vi "Main.vi"(8 "error in":errorcluster, 11 "TCP Receive in":refnum<class "TCP Receive.lvclass">) -> (0 "error out":errorcluster, 3 "TCP Receive out":refnum<class "TCP Receive.lvclass">)   [LabVIEW 2020, in "TCP Receive.lvclass"]
doc: "The Queued Message Handler of a Worker."
uses:
  TCP Receive.lvclass
  C:/Program Files (x86)/National Instruments/LabVIEW 2020/vi.lib/addons/_Workers/Library/Classes/Worker/Worker.lvclass
  Initialization Data.ctl
  <vilib>/addons/_Workers/Library/Classes/Message Queue/Message Queue.lvclass
  TCP Receive.lvclass/TCP Receive.ctl
  <vilib>/addons/_Workers/Library/Classes/Message/Enqueue Message to Self.vi
  <vilib>/addons/_Workers/Library/Classes/Message/Enqueue Message to Queue.vi
  <vilib>/addons/_Workers/Library/Classes/EHL/EHL.lvclass
  <vilib>/addons/_Workers/Library/Classes/Worker/Worker.lvclass
  <vilib>/addons/_Workers/Library/Classes/Error Handler/Error Handler.lvclass
  C:/Program Files (x86)/National Instruments/LabVIEW 2020/vi.lib/addons/_Workers/Library/Classes/Worker User/Worker User.lvclass
  C:/Program Files (x86)/National Instruments/LabVIEW 2020/vi.lib/addons/_Workers/Library/Classes/Workers Object/Workers Object.lvclass
  C:/Users/TestAdmin/git/TCP-Workers/Workers/TCP Receive/TCP Receive.lvclass
  <vilib>/addons/_Workers/Library/Classes/Message/Message.lvclass
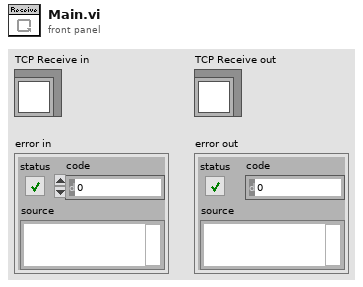
[diagram p1: front panel]
types:
  T1 = typedef "TCP Receive.lvclass/Initialization Data.ctl" = cluster{"String":string, "connection ID":refnum<k5>, "End Point":refnum<class "Message Queue.lvclass">}
  T2 = enum16{"Standard", "Buffered", "CRLF", "Immediate"}
  T3 = typedef "Workers.lvlib/Case Label.ctl" = string
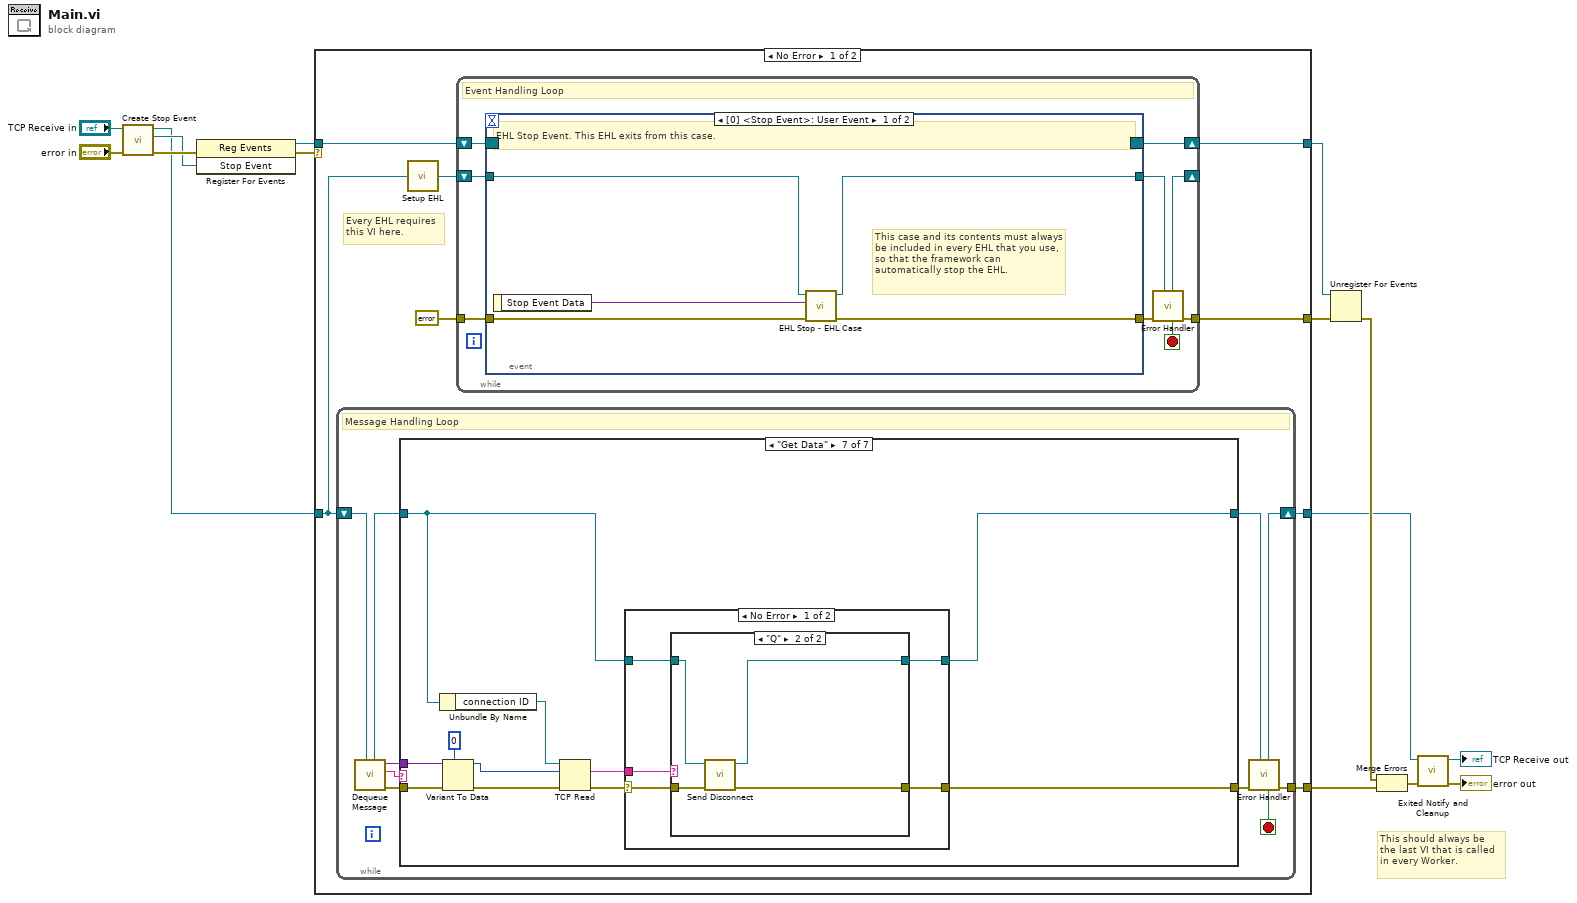
[diagram p0: block diagram]
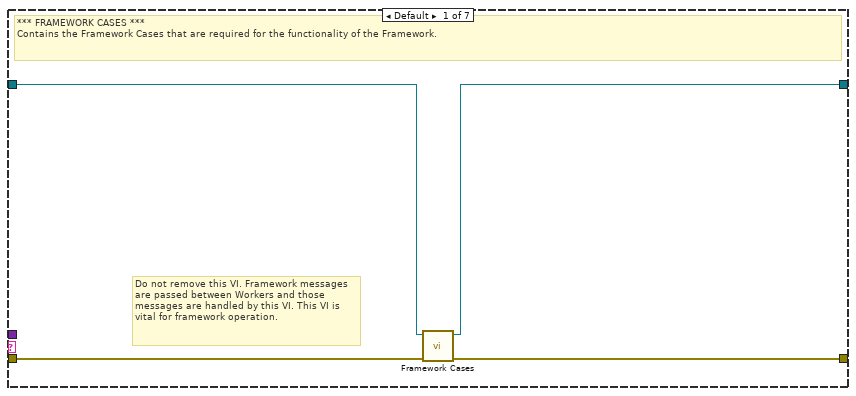
[diagram p2: hidden frame]
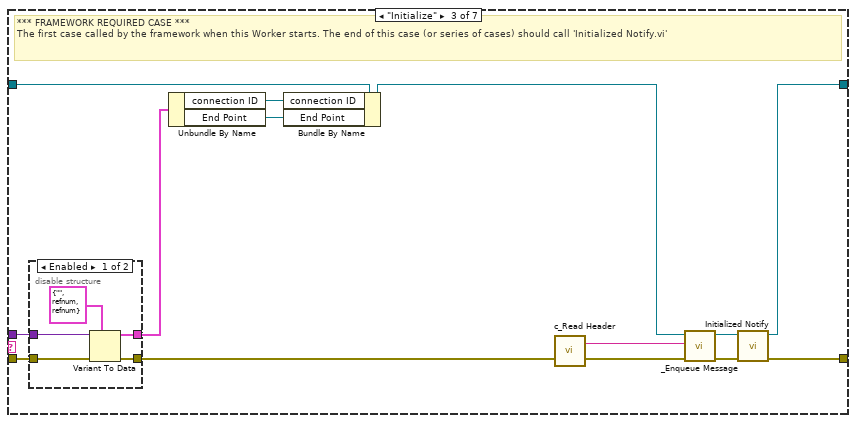
[diagram p4: hidden frame]
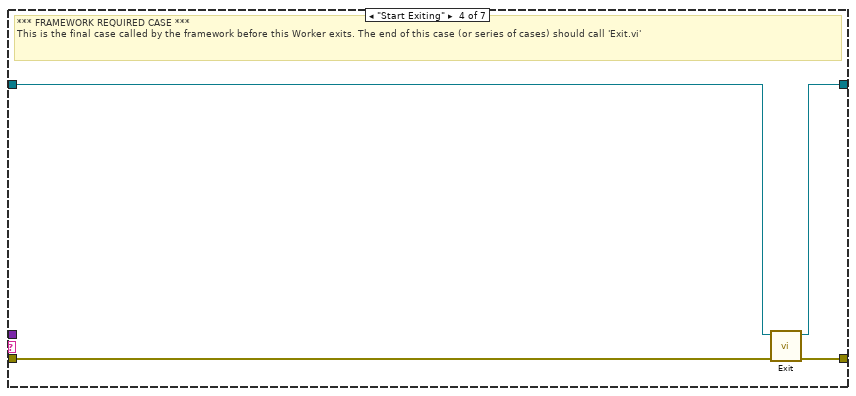
[diagram p6: hidden frame]
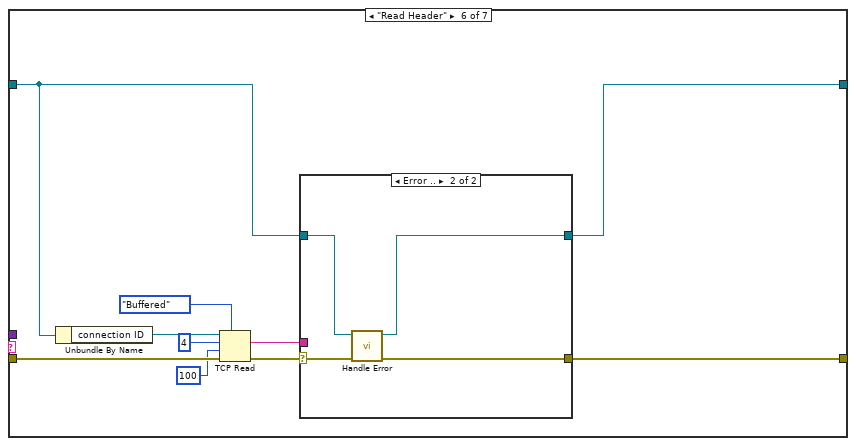
[diagram p8: hidden frame]
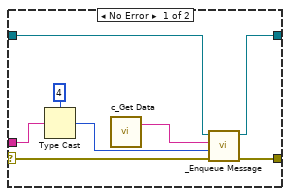
[diagram p9: hidden frame]
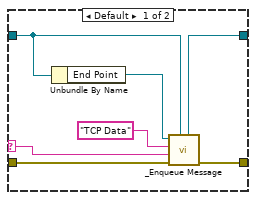
[diagram p10: hidden frame]
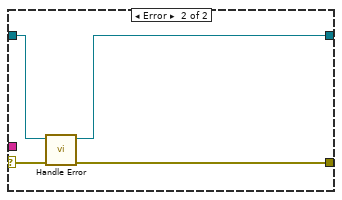
[diagram p11: hidden frame]
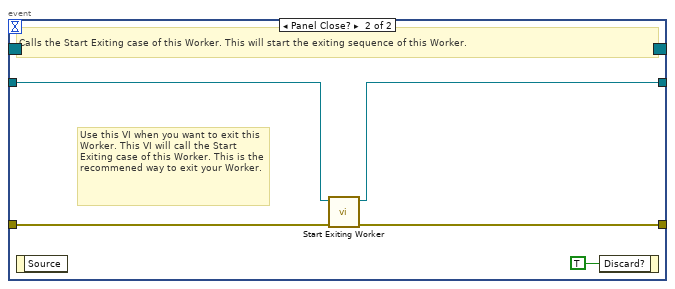
[diagram p12: hidden frame]
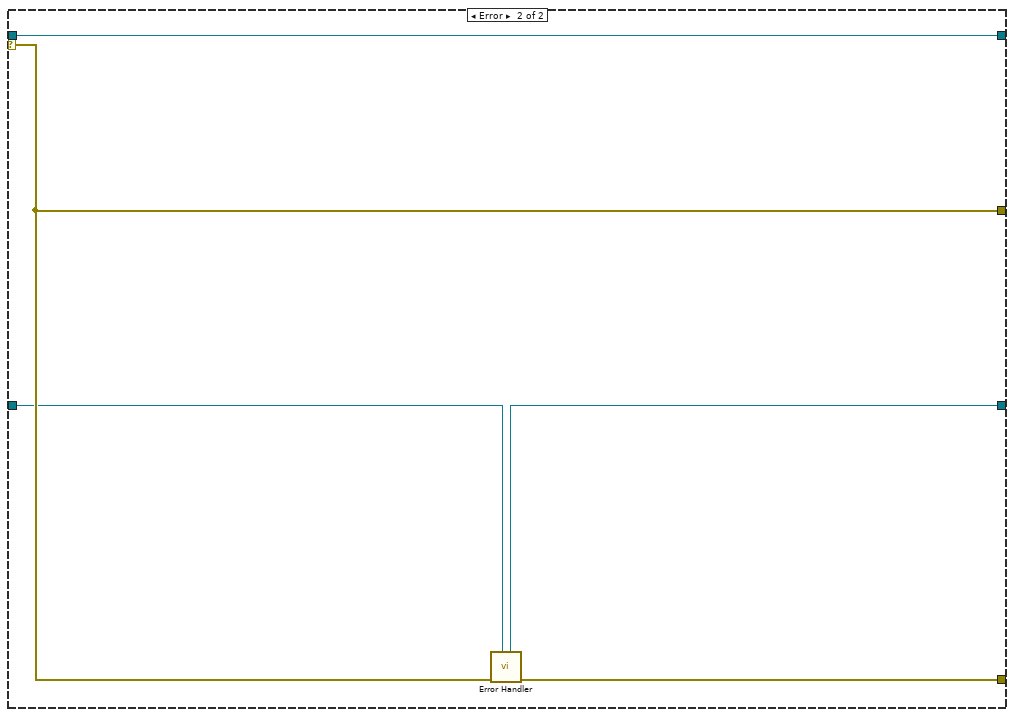
[diagram p13: hidden frame]
diagram:
  # "This should always be the last VI that is called in every Worker."
  n1 = call <vilib>:"Create Stop Event.vi"("error in"="error in", "Worker"="TCP Receive in") -> ("error out"=w10:errorcluster, "Stop Event"=w7:refnum<user-event>, "Worker out"=w4:refnum<class "TCP Receive.lvclass">)  [unwired: 7 in]
  n2 = register-events(error in=w10, w7) -> (reference out=w9:refnum<event-registration>, error out=w1:errorcluster)  [unwired: 1 in]
  n3 = case shown="No Error" w1 {
    tunnel: w4 -> [w18 w138]
    tunnel: [w16 w139] -> w8
    tunnel: w9 -> [w23 w140]
    tunnel: [w20 w141] -> w14
    tunnel: [w22 w140] -> w13
    tunnel: [w17 w137] -> w11
    selector: w1 -> [_ w141]
    frame No Error {
      # "Every EHL requires\nthis VI here."
      n4 = while {
        shift-right: [w31] -> w17
        shift-left: w18 -> [w33]
        tunnel: [w32] -> w16
        stop <- w24 stop-if-true
        # "Message Handling Loop"
        n5 = call <vilib>:"Dequeue Message.vi"("Worker"=w33) -> ("error out"=w30:errorcluster, "Case out"=w25:string, "Data out"=w26:variant, "Worker out"=w28:refnum<class "TCP Receive.lvclass">)  [unwired: 6 in, 1 out]
        n6 = case "WORKERS MHL Case Structure (DO NOT CHANGE LABEL NAME)" shown="\"Get Data\"" w25 {
          tunnel: w30 -> [w37 w38 w50 w59 w63 w74 w97]
          tunnel: [w36 w38 w52 w62 w63 w67 w88] -> w29
          tunnel: w28 -> [w35 w39 w49 w60 w64 w66 w89]
          tunnel: [w34 w39 w51 w61 w64 w65 w87] -> w27
          tunnel: w26 -> [_ _ w47 _ _ _ w95]
          frame Default {
            # "Do not remove this VI. Framework messages are passed between Workers and those messages are handled by this VI. This VI is vital for framework operation."
            # "*** FRAMEWORK CASES ***\nContains the Framework Cases that are required for the functionality of the Framework."
            n7 = call <vilib>:"Framework Cases.vi"("error in"=w37, "Worker"=w35) -> ("error out"=w36:errorcluster, "Worker out"=w34:refnum<class "TCP Receive.lvclass">)  [unwired: 8 in]
          }
          frame "------ FRAMEWORK REQUIRED CASES ------" {
            # "Start of Framework Required Cases"
          }
          frame "Initialize" {
            # "*** FRAMEWORK REQUIRED CASE ***\nThe first case called by the framework when this Worker starts. The end of this case (or series of cases) should call 'Initialized Notify.vi'"
            n8 = disable-structure shown="Enabled" {
              disable-tunnel: w50 -> [w57 w58]
              disable-tunnel: [w56 w58] -> w48
              disable-tunnel: w47 -> [w55 _]
              disable-tunnel: [w53 _] -> w46
              frame Enabled {
                n9 = Variant To Data(error in=w57, type=T1 {"String"="", "connection ID"=refnum, "End Point"=refnum} ("Initialization Data"), Variant=w55) -> (data=w53:T1, error out=w56:errorcluster)
              }
              frame Disabled {
              }
            }
            n10 = Unbundle By Name(w46) -> ("connection ID"=w45:refnum<k5>, "End Point"=w44:refnum<class "Message Queue.lvclass">)
            n11 = Bundle By Name(cluster=w49, "connection ID"=w45, "End Point"=w44) -> (w42:refnum<class "TCP Receive.lvclass">)
            n12 = call "c_Read Header.vi"() -> ("Case Label"=w40:T3)  [unwired: 1 in]
            n13 = call-poly <vilib>:"_Enqueue Message.vi"("error in"=w48, "Case Label"=w40, "Worker"=w42) -> ("error out"=w43:errorcluster, "dup Worker out"=w41:refnum<class "TCP Receive.lvclass">)  [unwired: 7 in]
            n14 = call <vilib>:"Initialized Notify.vi"("error in"=w43, "Worker"=w41) -> ("error out"=w52:errorcluster, "dup Worker out"=w51:refnum<class "TCP Receive.lvclass">)  [unwired: 8 in]
          }
          frame "Start Exiting" {
            # "*** FRAMEWORK REQUIRED CASE ***\nThis is the final case called by the framework before this Worker exits. The end of this case (or series of cases) should call 'Exit.vi'"
            n15 = call <vilib>:"Exit.vi"("error_in"=w59, "Worker"=w60) -> ("error out"=w62:errorcluster, "dup Worker out"=w61:refnum<class "TCP Receive.lvclass">)  [unwired: 8 in]
          }
          frame "-----------------------------------------------" {
            # "End of Framework Required Cases"
          }
          frame "Read Header" {
            n16 = Unbundle By Name(w66) -> ("connection ID"=w73:refnum<k5>)
            n17 = TCP Read(connection ID=w73, bytes to read=4, error in (no error)=w74, 7:T2."Buffered" ("mode (standard)"), 9:100 ("timeout ms (25000)")) -> (data out=w68:string, error out=w69:errorcluster)  [unwired: 1 out]
            n18 = case shown="Error .." w69 {
              selector: w69 -> [w80 w86]
              tunnel: w68 -> [w82 _]
              tunnel: [w77 w85] -> w67
              tunnel: w66 -> [w76 w84]
              tunnel: [w75 w83] -> w65
              frame No Error {
                n19 = Type Cast(type=4 ("bytes to read"), x=w82) -> (*(type *) &x=w79:i32)
                n20 = call "c_Get Data.vi"() -> ("Case Label"=w78:T3)  [unwired: 1 in]
                n21 = call-poly <vilib>:"_Enqueue Message.vi"("error in"=w80, "Data"=w79, "Case Label"=w78, "Worker"=w76) -> ("error out"=w77:errorcluster, "dup Worker out"=w75:refnum<class "TCP Receive.lvclass">)  [unwired: 6 in]
              }
              frame Error {
                n22 = call "Handle Error.vi"("error in (no error)"=w86, "TCP Receive in"=w84) -> ("error out"=w85:errorcluster, "TCP Receive out"=w83:refnum<class "TCP Receive.lvclass">)  [unwired: 8 in]
              }
            }
          }
          frame "Get Data" {
            n23 = Unbundle By Name(w89) -> ("connection ID"=w92:refnum<k5>)
            n24 = Variant To Data(error in=w97, type=0, Variant=w95) -> (data=w93:i32, error out=w96:errorcluster)
            n25 = TCP Read(connection ID=w92, bytes to read=w93, error in (no error)=w96) -> (data out=w90:string, error out=w91:errorcluster)  [unwired: 2 in, 1 out]
            n26 = case shown="No Error" w91 {
              selector: w91 -> [w102 w117]
              tunnel: w90 -> [w101 _]
              tunnel: w89 -> [w100 w116]
              tunnel: [w98 w115] -> w87
              tunnel: [w99 w114] -> w88
              frame No Error {
                n27 = case shown="\"Q\"" w101 {
                  selector: w101 -> [w104 _]
                  tunnel: w102 -> [w109 w113]
                  tunnel: w100 -> [w106 w111]
                  tunnel: [w108 w112] -> w99
                  tunnel: [w107 w110] -> w98
                  frame Default {
                    n28 = Unbundle By Name(w106) -> ("End Point"=w105:refnum<class "Message Queue.lvclass">)
                    n29 = call-poly <vilib>:"_Enqueue Message.vi"("Worker"=w106, "error in"=w109, "Data"=w104, "Case Label"="TCP Data", "Message Queue"=w105) -> ("error out"=w108:errorcluster, "dup Worker out"=w107:refnum<class "TCP Receive.lvclass">)  [unwired: 4 in, 1 out]
                  }
                  frame "Q" {
                    n30 = call "Send Disconnect.vi"("error in (no error)"=w113, "TCP Receive in"=w111) -> ("error out"=w112:errorcluster, "TCP Receive out"=w110:refnum<class "TCP Receive.lvclass">)  [unwired: 8 in]
                  }
                }
              }
              frame Error {
                n31 = call "Handle Error.vi"("error in (no error)"=w117, "TCP Receive in"=w116) -> ("error out"=w114:errorcluster, "TCP Receive out"=w115:refnum<class "TCP Receive.lvclass">)  [unwired: 8 in]
              }
            }
          }
        }
        n32 = call <vilib>:"Error Handler.vi"("Worker"=w27, "error_in"=w29) -> ("error out"=w32:errorcluster, "Stop Loop"=w24:bool, "Worker out"=w31:refnum<class "TCP Receive.lvclass">)  [unwired: 7 in]
      }
      n33 = call <vilib>:"Setup EHL.vi"("Worker"=w18) -> ("Worker out"=w19:refnum<class "TCP Receive.lvclass">)  [unwired: 14 in]
      n34 = while "Event Handling Loop" {
        shift-right: [w126] -> w22
        shift-left: w23 -> [w125]
        tunnel: [w121] -> w20
        tunnel: errorcluster {"status"=FALSE, "code"=0, "source"=""} ("error constant") -> [w123]
        shift-right: [w119] -> _
        shift-left: w19 -> [w124]
        stop <- w118 stop-if-true
        # "Event Handling Loop"
        n35 = event shown="[0] <Stop Event>: User Event" {
          selector: w125 -> [_ _]
          dyn-events: [_ _] -> w126
          timeout: _ -> [_ _]
          tunnel: [w130 w135] -> w122
          tunnel: w123 -> [w131 w134]
          tunnel: w124 -> [w129 w133]
          tunnel: [w128 w132] -> w120
          event User Event {
            # "This case and its contents must always be included in every EHL that you use, so that the framework can automatically stop the EHL."
            # "EHL Stop Event. This EHL exits from this case."
            n36 = event-data() -> ("Stop Event Data"=w127:variant)  [unwired: 1 in]
            n37 = call <vilib>:"EHL Stop - EHL Case.vi"("error in"=w131, "Stop Event Data"=w127, "Worker"=w129) -> ("error out"=w130:errorcluster, "Worker out"=w128:refnum<class "TCP Receive.lvclass">)  [unwired: 7 in]
          }
          event Panel Close? {
            # "Use this VI when you want to exit this Worker. This VI will call the Start Exiting case of this Worker. This is the recommened way to exit your Worker."
            # "Calls the Start Exiting case of this Worker. This will start the exiting sequence of this Worker."
            n38 = event-data() -> ()  [unwired: 1 in, 1 out]
            n39 = call <vilib>:"Start Exiting Worker.vi"("error in"=w134, "Worker"=w133) -> ("error out"=w135:errorcluster, "dup Worker out"=w132:refnum<class "TCP Receive.lvclass">)  [unwired: 8 in]
            n40 = event-data("Discard?"=TRUE) -> ()  [unwired: 1 in, 1 out]
          }
        }
        n41 = call <vilib>:"Error Handler.vi"("Worker"=w120, "error_in"=w122) -> ("error out"=w121:errorcluster, "Stop Loop"=w118:bool, "Worker out"=w119:refnum<class "TCP Receive.lvclass">)  [unwired: 7 in]
      }
    }
    frame Error {
      n42 = call <vilib>:"Error Handler.vi"("Worker"=w138, "error_in"=w141) -> ("error out"=w139:errorcluster, "Worker out"=w137:refnum<class "TCP Receive.lvclass">)  [unwired: 7 in, 1 out]
    }
  }
  n43 = Unregister For Events(event registration refnum=w13, error in=w14) -> (error out=w15:errorcluster)
  n44 = Merge Errors(w15, w8) -> (w12:errorcluster)
  n45 = call <vilib>:"Exited Notify and Cleanup.vi"("error_in"=w12, "Worker"=w11) -> ("error out"=→"error out":errorcluster, "dup Worker out"=→"TCP Receive out":refnum<class "TCP Receive.lvclass">)  [unwired: 8 in]
